vi "Read Measurement (Channel Power Measurement).vi"(0 "VISA resource name":refnum<visa-resource-name>, 5 "Timeout (10000 ms)":i32=10000 format="%.0g", 11 "error in (no error)":errorcluster) -> (4 "VISA resource name out":refnum<visa-resource-name>, 6 "Channel Power":dbl, 8 "Power Spectral Density":dbl, 15 "error out":errorcluster)   [LabVIEW 2018, in "Agilent MXA Series.lvlib"]
doc: "Reads the measurement result from the spectrum analyzer(Channel Power Measurement)."
uses:
  Agilent MXA Series.lvlib
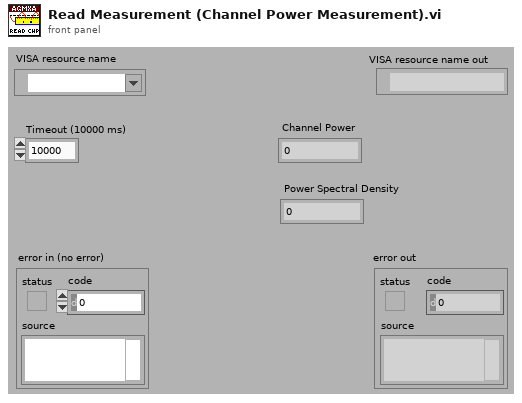
[diagram p1: front panel]
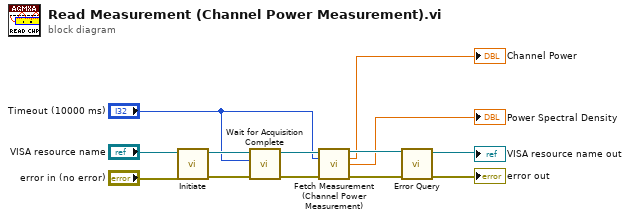
[diagram p0: block diagram]
diagram:
  n1 = call "Initiate.vi"("error in (no error)"="error in (no error)", "VISA resource name"="VISA resource name") -> ("error out"=w10:errorcluster, "VISA resource name out"=w11:refnum<visa-resource-name>)  [unwired: 8 in]
  n2 = call "Wait for Acquisition Complete.vi"("error in (no error)"=w10, "Maximum Time (10000)"="Timeout (10000 ms)", "VISA resource name"=w11) -> ("error out"=w8:errorcluster, "VISA resource name out"=w9:refnum<visa-resource-name>)  [unwired: 7 in]
  n3 = call "Fetch Measurement (Channel Power Measurement).vi"("VISA resource name"=w9, "Timeout (10000 ms)"="Timeout (10000 ms)", "error in (no error)"=w8) -> ("VISA resource name out"=w7:refnum<visa-resource-name>, "Channel Power"=→"Channel Power":dbl, "Power Spectral Density"=→"Power Spectral Density":dbl, "error out"=w6:errorcluster)  [unwired: 9 in]
  n4 = call "Error Query.vi"("error in (no error)"=w6, "VISA resource name"=w7) -> ("error out"=→"error out":errorcluster, "VISA resource name out"=→"VISA resource name out":refnum<visa-resource-name>)  [unwired: 6 in, 2 out]
